vi "test1.vi"() -> ()   [LabVIEW 2024]
uses:
  <vilib>/Instr/_visa.llb/VISA Find Search Mode.ctl
  <vilib>/Instr/_visa.llb/VISA Configure Serial Port (Instr).vi
panel:
  out "transmission time":dbl
  out "unsigned byte array":u8[](array[numeric])
  out "find list":string[](array[string])
  out "String":string
  in  "stop":bool
  in  "VISA Reciever":refnum<visa-resource-name>="ASRL1::INSTR"
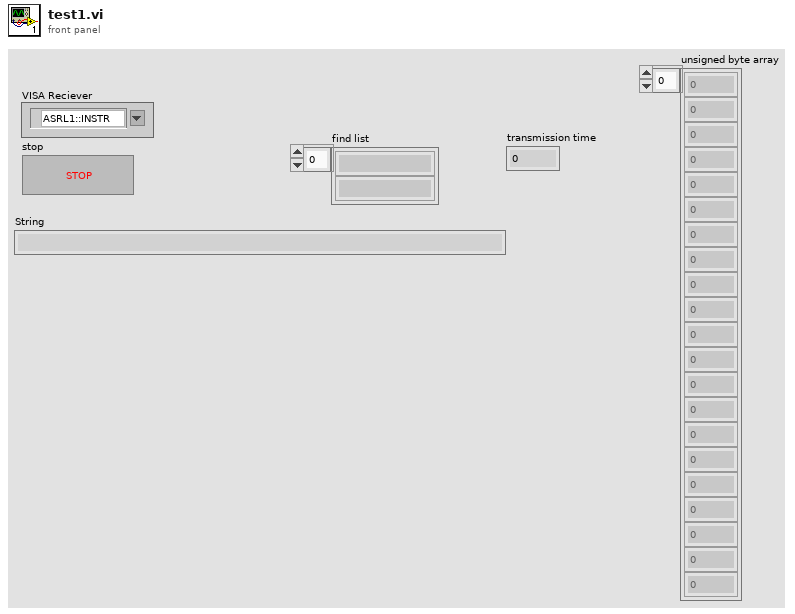
[diagram p1: front panel]
types:
  T1 = typedef "VISA Find Search Mode.ctl" = u32
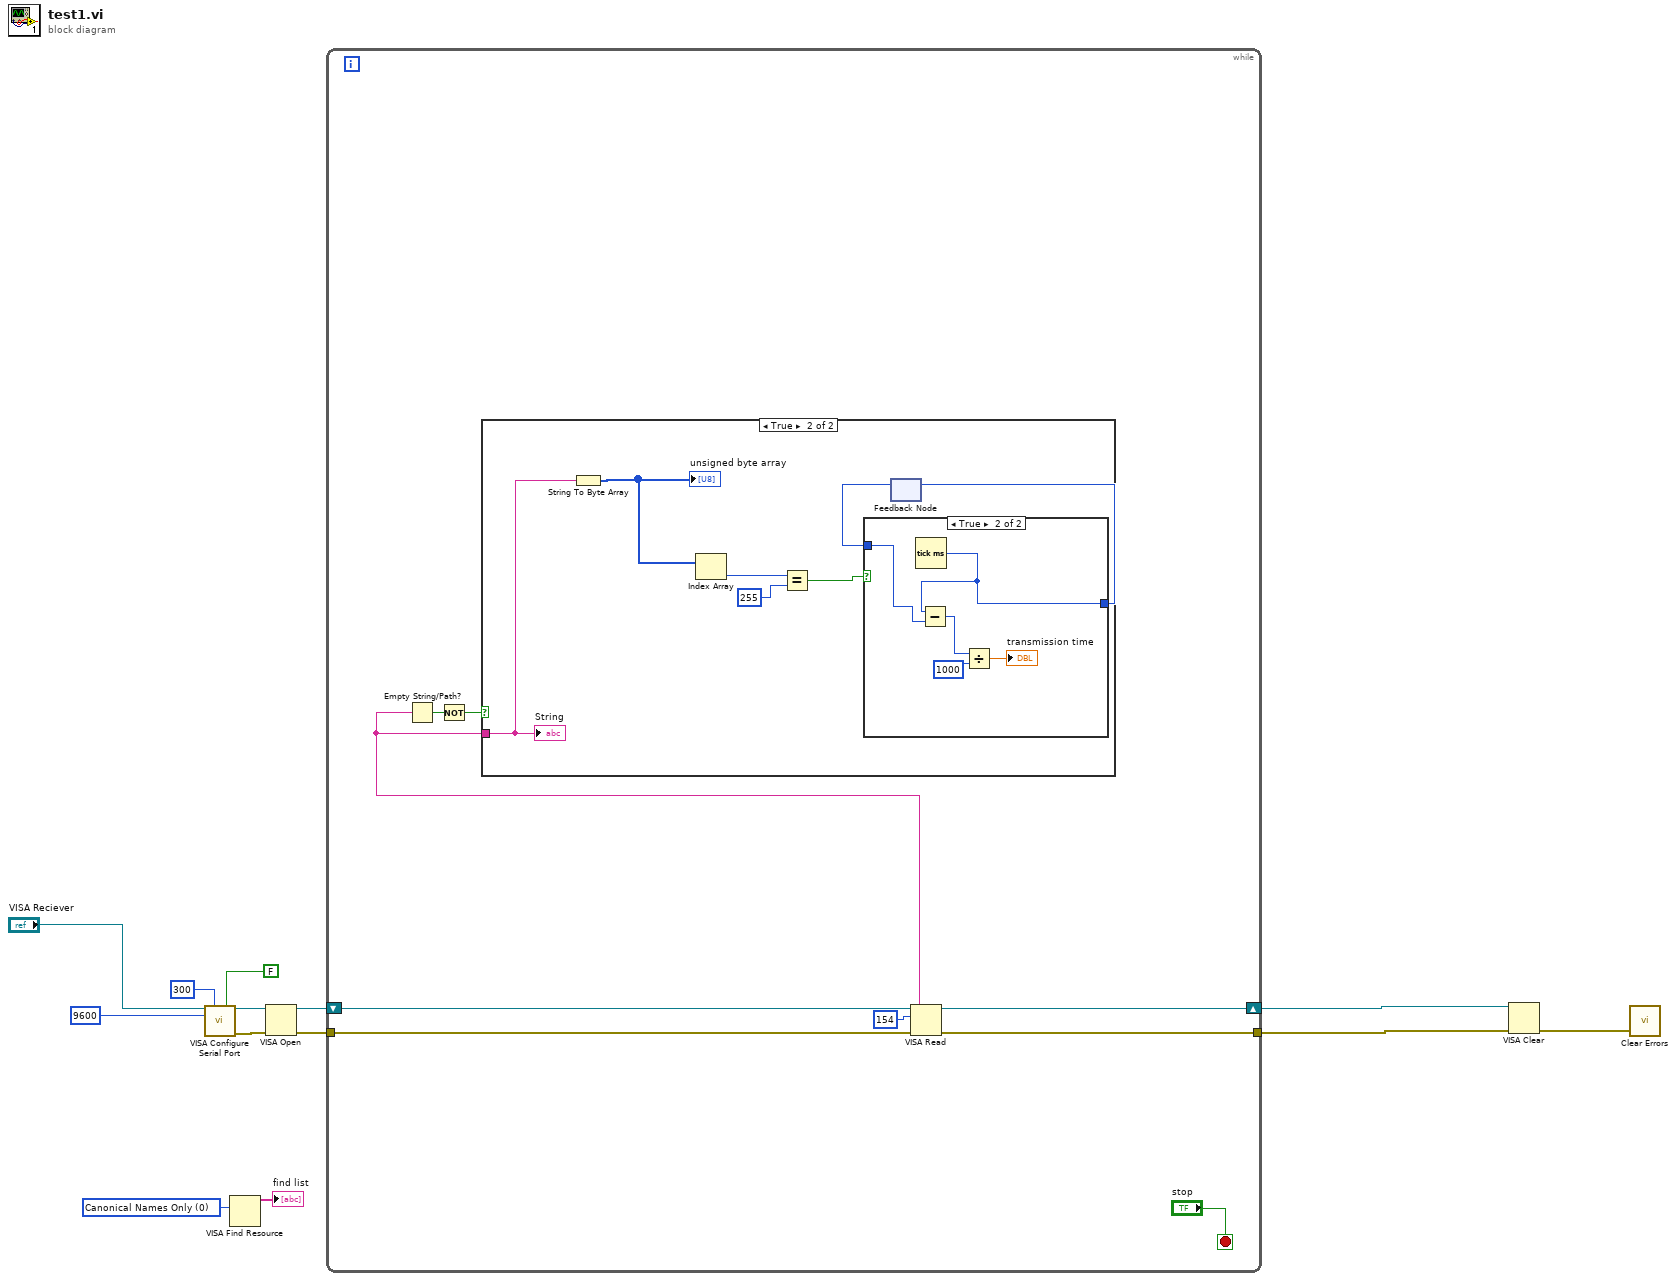
[diagram p0: block diagram]
diagram:
  w2 = T1 0 items=["Canonical Names Only"=0, "Aliases Only"=2, "Include Matching Aliases"=3, "Include All Aliases"=4] ("Search Mode")
  n1 = call-poly "VISA Configure Serial Port"("VISA resource name"="VISA Reciever", "timeout (10sec)"=u32 300, "Enable Termination\nChar (T)"=FALSE ("Enable Termination\nChar (T)"), "baud rate (9600)"=u32 9600) -> ("VISA resource name out"=w10:refnum<visa-resource-name>, "error out"=w7:errorcluster)  [unwired: 10 in]
  n2 = VISA Find Resource(10:w2) -> (3:→"find list":string[])  [unwired: 2 in, 2 out]
  n3 = VISA Open(error in (no error)=w7, VISA resource name=w10) -> (VISA resource name=w9:refnum<visa-resource-name>, error out=w8:errorcluster)  [unwired: 3 in]
  n4 = while {
    shift-right: [w21] -> w5
    shift-left: w9 -> [w19]
    tunnel: w8 -> [w14]
    tunnel: [w20] -> w4
    stop <- "stop" stop-if-true
    n5 = VISA Read(VISA resource name=w19, byte count=u32 154, error in (no error)=w14) -> (VISA resource name out=w21:refnum<visa-resource-name>, read buffer=w15:string, error out=w20:errorcluster)  [unwired: 1 out]
    n6 = Empty String/Path?(string/path=w15) -> (empty?=w18:bool)
    n7 = Not(x=w18) -> (.not. x?=w17:bool)
    n8 = case shown="True" w17 {
      tunnel: w15 -> [_ w29]
      frame False {
      }
      frame True {
        n9 = String To Byte Array(string=w29) -> (unsigned byte array=w28:u8[])
        "unsigned byte array" <- w28
        n10 = Index Array(array=w28) -> (element=w27:u8)  [unwired: 1 in]
        n11 = Equal?(x=w27, y=u8 255) -> (x = y?=w23:bool)
        n12 = feedback #1() -> (w24:u32)  [unwired: 1 in]
        n13 = case shown="True" w23 {
          tunnel: [w30 w35] -> w25
          tunnel: w24 -> [w30 w34]
          frame False {
          }
          frame True {
            n14 = Tick Count (ms)() -> (millisecond timer value=w35:u32)
            n15 = Subtract(x=w35, y=w34) -> (x-y=w33:u32)
            n16 = Divide(x=w33, y=u32 1000) -> (x/y=→"transmission time":dbl)
          }
        }
        n17 = feedback-in #1(w25) -> ()
        "String" <- w29
      }
    }
  }
  n18 = VISA Clear(VISA resource name=w5, error in (no error)=w4) -> (error out=w6:errorcluster)  [unwired: 1 out]
  n19 = call <vilib>:"Clear Errors.vi"("error in (no error)"=w6) -> ()  [unwired: 5 in, 2 out]
